vi "Get Tag Object.vi"(8 "error in (no error)":errorcluster, 9 "Coords (if tag empty)":T1, 10 "Tag (string)":string, 11 "Tree_LVOOP in":refnum<class "Tree Class.lvclass">) -> (0 "error out":errorcluster, 1 "InGlyph":bool, 2 "Tag":refnum<class "Tree Tag Class.lvclass">, 3 "Tree_LVOOP out":refnum<class "Tree Class.lvclass">)   [LabVIEW 2012, in "Tree Tools.lvlib" / "Tree Class.lvclass"]
uses:
  Tree Class.lvclass
  <vilib>/Utility/miscctls.llb/LVPoint32TypeDef.ctl
  Tree Tag Class/Tree Tag Class.lvclass
  Tree Class.lvclass/Tree Class.ctl
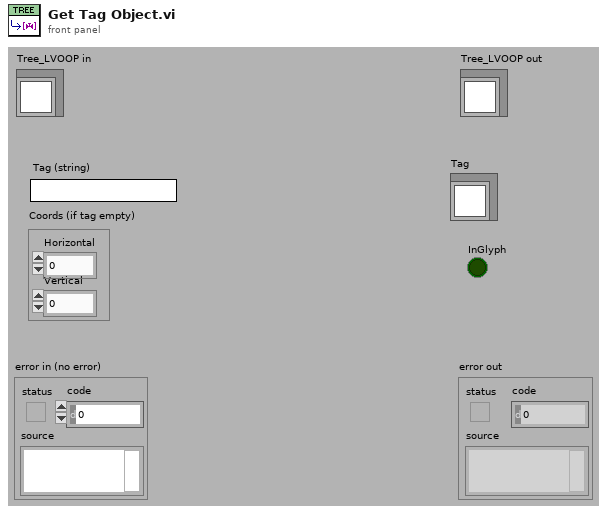
[diagram p1: front panel]
types:
  T1 = typedef "LVPoint32TypeDef.ctl" = cluster{"Horizontal":i32, "Vertical":i32}
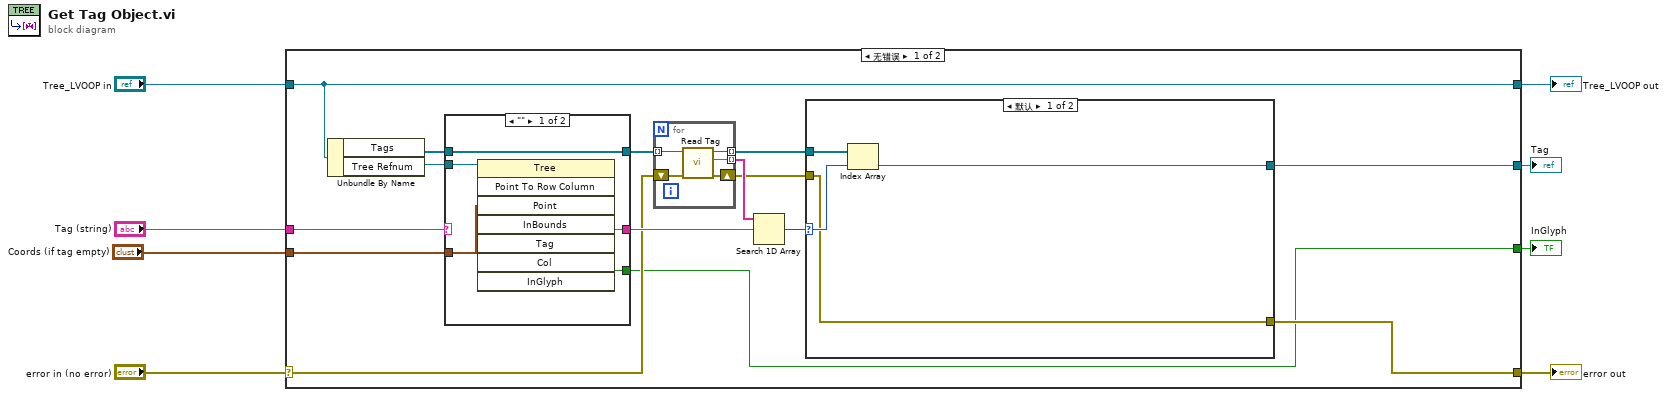
[diagram p0: block diagram]
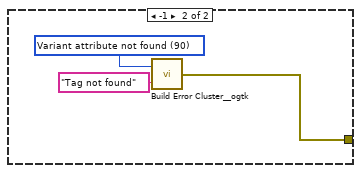
[diagram p2: hidden frame]
diagram:
  n1 = case shown="无错误" "error in (no error)" {
    selector: "error in (no error)" -> [w11 w44]
    tunnel: [w10 w44] -> w7
    tunnel: [w23 w43] -> w5
    tunnel: "Tree_LVOOP in" -> [w23 w43]
    tunnel: "Tag (string)" -> [w21 _]
    tunnel: "Coords (if tag empty)" -> [w19 _]
    tunnel: [w13 _] -> w2
    tunnel: [w9 _] -> w1
    frame No Error {
      n2 = Unbundle By Name(w23) -> ("Tags"=w22:refnum<class "Tree Tag Class.lvclass">[], "Tree Refnum"=w20:refnum<vi>)
      n3 = case shown="\"\"" w21 {
        selector: w21 -> [_ w42]
        tunnel: w22 -> [w37 w41]
        tunnel: w20 -> [w40 _]
        tunnel: w19 -> [w39 _]
        tunnel: [w38 w42] -> w16
        tunnel: [w37 w41] -> w17
        tunnel: [w36 _] -> w9
        frame "" {
          n4 = invoke class="Tree" method="Point To Row Column"(reference=w40, "Point"=w39) -> ("Tag"=w38:string, "InGlyph"=w36:bool)  [unwired: 6 in, 6 out]
        }
        frame Default {
        }
      }
      n5 = for {
        tunnel: w17 -> [w35] mode=indexing
        tunnel: [w34] -> w18 mode=indexing
        tunnel: [w33] -> w14 mode=indexing
        shift-right: [w31] -> w12
        shift-left: w11 -> [w32]
        n6 = call-dynamic "Read Tag.vi"("error in (no error)"=w32, "Tag_LVOOP.lvclass in"=w35) -> ("error out"=w31:errorcluster, "Tag"=w34:string, "Tag_LVOOP.lvclass out"=w33:refnum<class "Tree Tag Class.lvclass">)  [unwired: 7 in]
      }
      n7 = Search 1D Array(1D array=w18, element=w16) -> (index of element=w15:i32)  [unwired: 1 out]
      n8 = case shown="默认" w15 {
        selector: w15 -> [w26 _]
        tunnel: w14 -> [w27 _]
        tunnel: [w25 _] -> w13
        tunnel: w12 -> [w24 _]
        tunnel: [w24 w29] -> w10
        frame Default {
          n9 = Index Array(array=w27, index=w26) -> (element=w25:refnum<class "Tree Tag Class.lvclass">)
        }
        frame -1 {
          w30 = 90 items=["No error", "Argument error", "Memory is full", "Out of zone", "End of file", "File already open", "Generic file I/O error", "File not found", "File permission error", "Disk is full", "Duplicate path", "Too many files open", "System feature not enabled", "Resource file not found", "Cannot add resource", "Resource not found", "Image not found", "Image memory error", "Pen does not exist", "Config type invalid", "Config token not found", "Config parse error", "Config memory error", "Bad external code format", "Bad external code offset", "External code not present", "Null window", "Destroy window error", "Null menu", "Print aborted", "Bad print record", "Print driver error", "Windows error during printing", "Memory error during printing", "Print dialog error", "Generic print error", "Invalid device refnum", "Device not found", "Device parameter error", "Device unit error", "Cannot open device", "Device call aborted", "Generic error", "Cancelled by user", "Object ID too low", "Object ID too high", "Object not in heap", "Unknown heap", "Unknown object (invalid DefProc)", "Unknown object (DefProc not in table)", "Message out of range", "Invalid (null) method", "Unknown message", "Manager call not supported", "Bad address", "Network operation in progress", "Network operation timed out", "Connection is busy", "Network attribute not supported", "Network error", "Address in use", "System out of memory", "Connection aborted", "Connection refused", "Not connected", "Already connected", "Connection closed", "Initialization error (interapplication manager)", "Bad occurrence", "Wait on unbound occurrence handler", "Occurrence queue overflow", "Datalog type conflict", "Unused", "Unrecognized type (interapplication manager)", "Memory corrupt", "Failed to make temporary DLL", "Old CIN version", "Drag socket not found", "Failed to load drop-object", "Failed to register OLE object", "Failed to release OLE object", "Format specifier type mismatch", "Unknown format specifier", "Too few format specifiers", "Too many format specifiers", "Scan failed", "Newer CIN version", "Error converting to variant", "Runtime menu error", "Password tampered", "Variant attribute not found", "Incompatible variant data type", "Event data is not available", "Event Store is not present", "Occurrence is not found", "Event Queue is not created", "Event info is not available", "Refnum passed is NULL", "Error retrieving Class GUID", "Error retrieving CoClass GUID", "Error retrieving TypeLib GUID.", "Bad built application magic bytes.", "Specific driver is different from the specific driver associated with the Logical Name.", "There is no session opened to the class driver.", "Max Error", "MAX - Error with config objects", "MAX - Error loading configuration", "MAX - Group not supported"]
          n10 = call <userlib>:"Build Error Cluster__ogtk.vi"("String to Prepend to source (\"\")"="Tag not found" ("String to Prepend to source (\"\")"), "code"=w30) -> ("error out"=w29:errorcluster)
        }
      }
    }
    frame Error {
    }
  }
  "error out" <- w7
  "Tree_LVOOP out" <- w5
  "Tag" <- w2
  "InGlyph" <- w1
